vi "CreateMaze.vi"(8 "error in (no error)":errorcluster, 11 "MazeGame in":refnum<class "MazeGame.lvclass">) -> (0 "error out":errorcluster, 2 "Maze*":refnum<data-value>, 3 "MazeGame out":refnum<class "MazeGame.lvclass">)   [LabVIEW 2016, in "MazeGame.lvclass"]
uses:
  MazeGame.lvclass
  Maze/Maze.lvclass
  Room/Direction.ctl
  Wall/Wall.lvclass
  C:/github/LVOOP-creational-patterns/Maze-Classes/src/MapSite/MapSite.lvclass
  Door/Door.lvclass
  Room/Room.lvclass
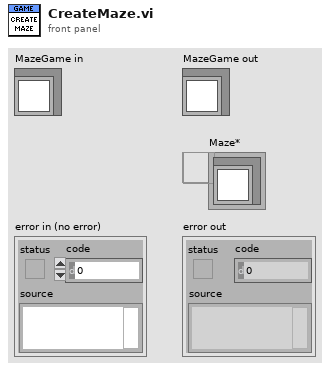
[diagram p1: front panel]
types:
  T1 = typedef "Room.lvclass/Direction.ctl" = enum16{"North", "South", "East", "West"}
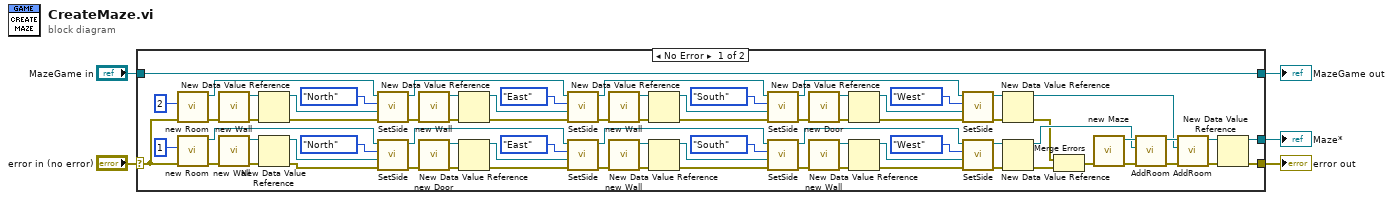
[diagram p0: block diagram]
diagram:
  n1 = case shown="No Error" "error in (no error)" {
    selector: "error in (no error)" -> [w7 w84]
    tunnel: [w6 w84] -> w4
    tunnel: [w82 w83] -> w2
    tunnel: "MazeGame in" -> [w82 w83]
    tunnel: [w72 _] -> w1
    frame No Error {
      n2 = call "new Room.vi"("error in (no error)"=w7, "roomNumber"=2) -> ("error out"=w21:errorcluster, "Room out"=w39:refnum<class "Room.lvclass">)  [unwired: 8 in]
      n3 = call "new Room.vi"("error in (no error)"=w7, "roomNumber"=1) -> ("error out"=w46:errorcluster, "Room out"=w71:refnum<class "Room.lvclass">)  [unwired: 8 in]
      n4 = call "new Wall.vi"("error in (no error)"=w21) -> ("error out"=w20:errorcluster, "Wall out"=w38:refnum<class "Wall.lvclass">)  [unwired: 9 in]
      n5 = call "new Wall.vi"("error in (no error)"=w46) -> ("error out"=w45:errorcluster, "Wall out"=w70:refnum<class "Wall.lvclass">)  [unwired: 9 in]
      n6 = New Data Value Reference(data value=w38, error in=w20) -> (data value reference=w37:refnum<data-value>, error out=w19:errorcluster)
      n7 = New Data Value Reference(data value=w70, error in=w45) -> (data value reference=w69:refnum<data-value>, error out=w44:errorcluster)
      n8 = call-dynamic "SetSide.vi"("error in (no error)"=w19, "MapSite*"=w37, "Direction"=Direction."North", "Room in"=w39) -> ("error out"=w15:errorcluster, "Room out"=w35:refnum<class "Room.lvclass">)  [unwired: 6 in]
      n9 = call-dynamic "SetSide.vi"("error in (no error)"=w44, "MapSite*"=w69, "Direction"=Direction."North", "Room in"=w71) -> ("error out"=w54:errorcluster, "Room out"=w67:refnum<class "Room.lvclass">)  [unwired: 6 in]
      n10 = call "new Wall.vi"("error in (no error)"=w15) -> ("error out"=w22:errorcluster, "Wall out"=w27:refnum<class "Wall.lvclass">)  [unwired: 9 in]
      n11 = call "new Door.vi"("error in (no error)"=w54) -> ("error out"=w80:errorcluster, "Door out"=w79:refnum<class "Door.lvclass">)  [unwired: 9 in]
      n12 = New Data Value Reference(data value=w27, error in=w22) -> (data value reference=w16:refnum<data-value>, error out=w14:errorcluster)
      n13 = New Data Value Reference(data value=w79, error in=w80) -> (data value reference=w59:refnum<data-value>, error out=w53:errorcluster)
      n14 = call-dynamic "SetSide.vi"("error in (no error)"=w14, "MapSite*"=w16, "Direction"=Direction."East", "Room in"=w35) -> ("error out"=w24:errorcluster, "Room out"=w34:refnum<class "Room.lvclass">)  [unwired: 6 in]
      n15 = call-dynamic "SetSide.vi"("error in (no error)"=w53, "MapSite*"=w59, "Direction"=Direction."East", "Room in"=w67) -> ("error out"=w52:errorcluster, "Room out"=w66:refnum<class "Room.lvclass">)  [unwired: 6 in]
      n16 = call "new Wall.vi"("error in (no error)"=w24) -> ("error out"=w18:errorcluster, "Wall out"=w26:refnum<class "Wall.lvclass">)  [unwired: 9 in]
      n17 = call "new Wall.vi"("error in (no error)"=w52) -> ("error out"=w51:errorcluster, "Wall out"=w57:refnum<class "Wall.lvclass">)  [unwired: 9 in]
      n18 = New Data Value Reference(data value=w26, error in=w18) -> (data value reference=w25:refnum<data-value>, error out=w23:errorcluster)
      n19 = New Data Value Reference(data value=w57, error in=w51) -> (data value reference=w56:refnum<data-value>, error out=w50:errorcluster)
      n20 = call-dynamic "SetSide.vi"("error in (no error)"=w23, "MapSite*"=w25, "Direction"=Direction."South", "Room in"=w34) -> ("error out"=w13:errorcluster, "Room out"=w32:refnum<class "Room.lvclass">)  [unwired: 6 in]
      n21 = call-dynamic "SetSide.vi"("error in (no error)"=w50, "MapSite*"=w56, "Direction"=Direction."South", "Room in"=w66) -> ("error out"=w49:errorcluster, "Room out"=w64:refnum<class "Room.lvclass">)  [unwired: 6 in]
      n22 = call "new Door.vi"("error in (no error)"=w13) -> ("error out"=w41:errorcluster, "Door out"=w40:refnum<class "Door.lvclass">)  [unwired: 9 in]
      n23 = call "new Wall.vi"("error in (no error)"=w49) -> ("error out"=w48:errorcluster, "Wall out"=w58:refnum<class "Wall.lvclass">)  [unwired: 9 in]
      n24 = New Data Value Reference(data value=w40, error in=w41) -> (data value reference=w17:refnum<data-value>, error out=w12:errorcluster)
      n25 = New Data Value Reference(data value=w58, error in=w48) -> (data value reference=w55:refnum<data-value>, error out=w47:errorcluster)
      n26 = call-dynamic "SetSide.vi"("error in (no error)"=w12, "MapSite*"=w17, "Direction"=Direction."West", "Room in"=w32) -> ("error out"=w33:errorcluster, "Room out"=w31:refnum<class "Room.lvclass">)  [unwired: 6 in]
      n27 = call-dynamic "SetSide.vi"("error in (no error)"=w47, "MapSite*"=w55, "Direction"=Direction."West", "Room in"=w64) -> ("error out"=w65:errorcluster, "Room out"=w63:refnum<class "Room.lvclass">)  [unwired: 6 in]
      n28 = New Data Value Reference(data value=w31, error in=w33) -> (data value reference=w11:refnum<data-value>, error out=w10:errorcluster)
      n29 = New Data Value Reference(data value=w63, error in=w65) -> (data value reference=w77:refnum<data-value>, error out=w9:errorcluster)
      n30 = Merge Errors(w10, w9) -> (w8:errorcluster)
      n31 = call "new Maze.vi"("error in (no error)"=w8) -> ("error out"=w43:errorcluster, "Maze out"=w78:refnum<class "Maze.lvclass">)  [unwired: 9 in]
      n32 = call-dynamic "AddRoom.vi"("error in (no error)"=w43, "Room*"=w77, "Maze in"=w78) -> ("error out"=w76:errorcluster, "Maze out"=w75:refnum<class "Maze.lvclass">)  [unwired: 7 in]
      n33 = call-dynamic "AddRoom.vi"("error in (no error)"=w76, "Room*"=w11, "Maze in"=w75) -> ("error out"=w74:errorcluster, "Maze out"=w73:refnum<class "Maze.lvclass">)  [unwired: 7 in]
      n34 = New Data Value Reference(data value=w73, error in=w74) -> (data value reference=w72:refnum<data-value>, error out=w6:errorcluster)
    }
    frame Error {
    }
  }
  "error out" <- w4
  "MazeGame out" <- w2
  "Maze*" <- w1
